vi "Get_Connect_Status.vi"(5 "Device Number":T1, 7 "Update":bool, 11 "Connected":bool) -> (3 "Connected":bool)   [LabVIEW 2016]
uses:
  _TypeDefs/FRIC_navX_DeviceNumbersTypeDef.ctl
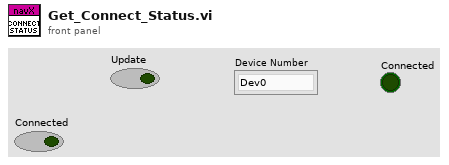
[diagram p1: front panel]
types:
  T1 = typedef "FRIC_navX_DeviceNumbersTypeDef.ctl" = enum16{"Dev0", "Dev1", "Dev2", "Dev3", "Dev4", "Dev5", "Dev6", "Dev7", "Dev8", "Dev9", "Dev10"}
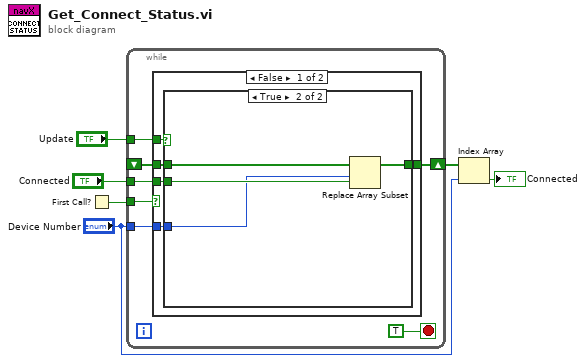
[diagram p0: block diagram]
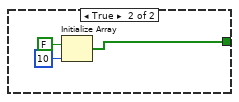
[diagram p3: hidden frame]
diagram:
  n1 = First Call?() -> (First Call?: T/F=w4:bool)
  n2 = while {
    tunnel: "Update" -> [w12]
    shift-right: [w9] -> w3
    shift-left: _ -> [w11]
    tunnel: "Connected" -> [w10]
    tunnel: w4 -> [w8]
    tunnel: "Device Number" -> [w7]
    stop <- TRUE stop-if-true
    n3 = case shown="False" w8 {
      tunnel: w12 -> [w18 _]
      tunnel: w11 -> [w17 _]
      tunnel: w10 -> [w16 _]
      tunnel: [w15 w24] -> w9
      tunnel: w7 -> [w14 _]
      frame False {
        n4 = case shown="True" w18 {
          tunnel: w17 -> [w19 w23]
          tunnel: w16 -> [_ w21]
          tunnel: [w19 w22] -> w15
          tunnel: w14 -> [_ w20]
          frame False {
          }
          frame True {
            n5 = Replace Array Subset(array=w23, new element=w21, index=w20) -> (w22:bool[])
          }
        }
      }
      frame True {
        n6 = Initialize Array(FALSE ("Connected"), 10 ("dimension size")) -> (w24:bool[])
      }
    }
  }
  n7 = Index Array(array=w3, index="Device Number") -> (element=→"Connected":bool)
